vi "From Veristand Master To Modbus.vi"(7 "Parameters":T1={"Interface Data"={"Name"="", "Unit ID"=0, "Refresh Rate"=0, "Write Rate"=0, "Write Mode"=enum."Value Change", "Interface Type"=enum."TCP Master", "TCP Settings"={"Address"="", "Port"=0, "Timeout"=0}, "Serial Settings"={"VISA resource name"="", "baud rate"=0, "parity (even)"=0, "flow control (none)"=0, "serial type"=enum."RTU", "Wire Mode"=-1}}, "Modbus Input Groups"=[], "Modbus Output Groups"=[], "error in (no error)"={"status"=FALSE, "code"=0, "source"=""}, "Modbus Input Engine Group Names"=[], "Modbus Output Engine Group Names"=[]} {"Interface Data"."Serial Settings"."Wire Mode" items=["Unknown"=-1, "RS485/Wire4"=0, "RS485/Wire2-EchoDTR"=1, "RS485/Wire2-CtrlDTR"=2, "RS485/Wire2-Auto"=3, "RS232/DTE"=128, "RS232/DCE"=129, "RS232/AUTO"=130]; "Interface Data"."Serial Settings"."parity (even)" items=["None", "Odd", "Even", "Mark", "Space"]; "Interface Data"."Serial Settings"."flow control (none)" items=["None", "XON/XOFF", "RTS/CTS", "XON/XOFF & RTS/CTS", "DTR/DSR", "XON/XOFF & DTR/DSR"]}, 8 "error in (no error)":errorcluster, 10 "Process in":refnum<class "Process.lvclass">, 11 "Modbus Master in":refnum<class "Modbus Master.lvclass">) -> ()   [LabVIEW 2020, in "Modbus Master Engine.lvlib"]
uses:
  Modbus Master Engine.lvlib
  <vilib>/NI/NIVS Inline Async API/_VS Inline Async API/Process/Process.lvclass
  Shared/Device Info.ctl
  Shared/Write Mode.ctl
  Shared/Controls/Interface Type.ctl
  Shared/Controls/Data Model/TCP Settings.ctl
  Shared/Controls/Data Model/Serial Settings.ctl
  Bulk Data Access.ctl
  System Explorer/SubVIs/Modbus Type.ctl
  Shared/Controls/Data Model/Channel.ctl
  <vilib>/NI VeriStand/Custom Device API/Custom Device Channel Type.ctl
  Shared/Controls/Data Model/Mapping.ctl
  Shared/Controls/Data Model/DataType.ctl
  <vilib>/NI VeriStand/Custom Device API/Custom Device Item Ref.ctl
  Includes/Modbus API.lvlibp/API/Master/Modbus Master.lvclass
  <vilib>/NI/NIVS Inline Async API/_Data Access Engine/Access Type Classes/Read/Read.lvclass/Read.ctl
  <vilib>/NI/NIVS Inline Async API/_VS Inline Async API/Process/Process.lvclass/Process.ctl
  <vilib>/NI/NIVS Inline Async API/_Data Access Engine/Data Access Engine/Methods/Read.Data.vi
  <vilib>/NI/NIVS Inline Async API/_VS Inline Async API/Error Handling Process/SubVIs/Error.ConvertArray.vi
  <vilib>/NI/NIVS Inline Async API/_Data Access Engine/Access Type Classes/Read/Read.ProcessData.vi
  <vilib>/NI/NIVS Inline Async API/_Data Access Engine/Data Access Engine/Data Access Engine.lvclass
  <vilib>/NI VeriStand/Custom Device Tools/Custom Device Utility Library/Custom Device Utility Library.lvlib
  <vilib>/NI/NIVS Inline Async API/_Data Access Engine/Access Type Classes/Write/Write.lvclass
  <vilib>/NI/NIVS Inline Async API/_Data Access Engine/Access Type Classes/Read/Read.lvclass
  Shared/Modbus Master Shared.lvlib
  <vilib>/NI VeriStand/Custom Device API/Custom Device API.lvlib
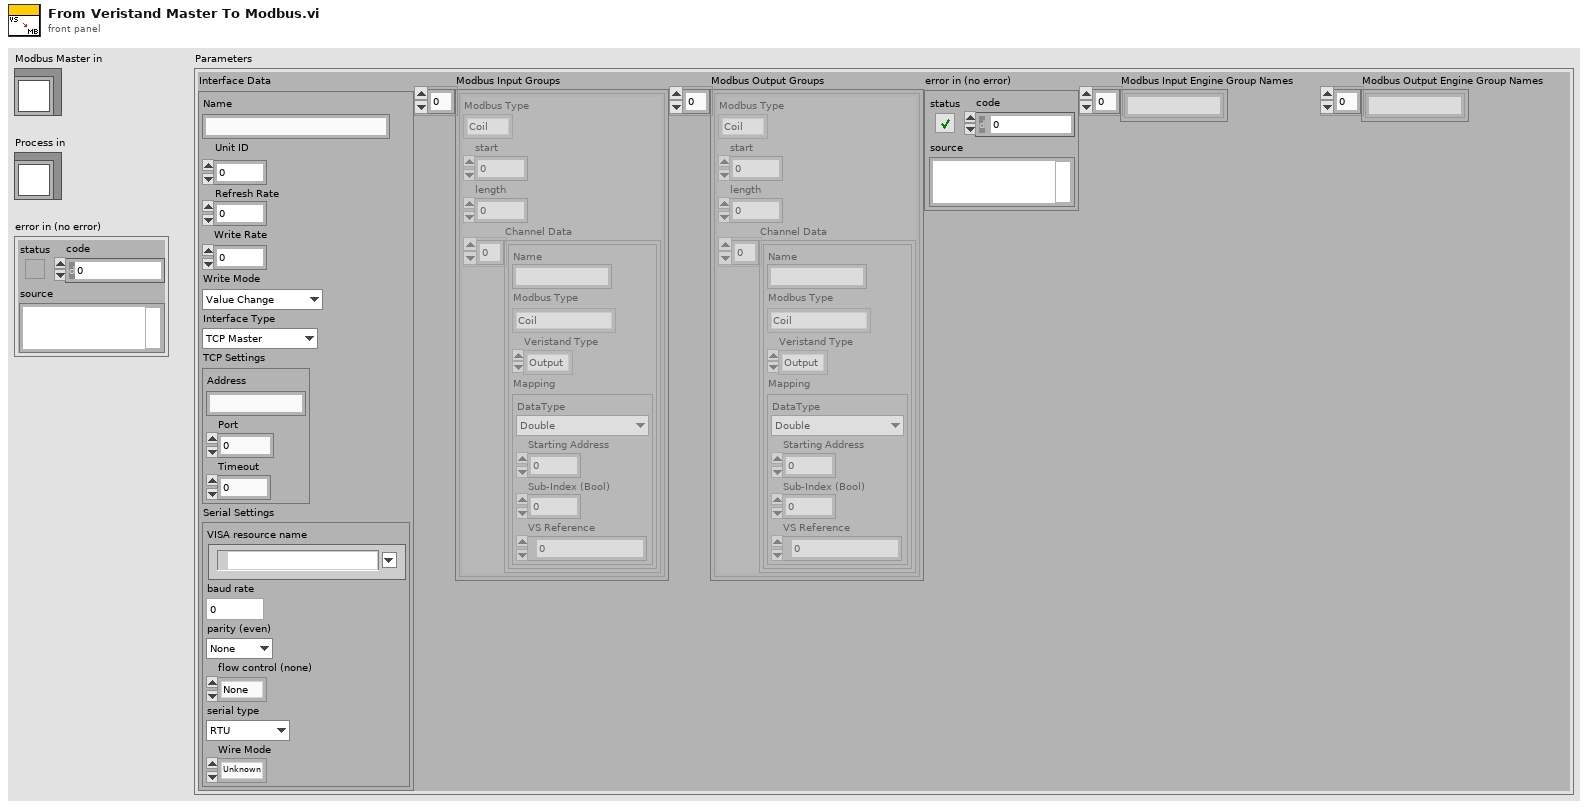
[diagram p1: front panel]
types:
  T1 = typedef "Modbus Master Shared.lvlib/Device Info.ctl" = cluster{"Interface Data":cluster{"Name":string, "Unit ID":u8, "Refresh Rate":i32, "Write Rate":i32, "Write Mode":T2, "Interface Type":T3, "TCP Settings":T4, "Serial Settings":T5}, "Modbus Input Groups":T6[], "Modbus Output Groups":T6[], "error in (no error)":errorcluster, "Modbus Input Engine Group Names":string[], "Modbus Output Engine Group Names":string[]}
  T2 = typedef "Modbus Master Shared.lvlib/Write Mode.ctl" = enum16{"Value Change", "Interval"}
  T3 = typedef "Modbus Master Shared.lvlib/Interface Type.ctl" = enum16{"TCP Master", "Serial Master", "TCP Slave", "Serial Slave"}
  T4 = typedef "Modbus Master Shared.lvlib/TCP Settings.ctl" = cluster{"Address":string, "Port":u16, "Timeout":i32}
  T5 = typedef "Modbus Master Shared.lvlib/Serial Settings.ctl" = cluster{"VISA resource name":refnum<visa-resource-name>, "baud rate":u32, "parity (even)":u16, "flow control (none)":u16, "serial type":enum16{"RTU", "ASCII"}, "Wire Mode":i16}
  T6 = typedef "Modbus Master Shared.lvlib/Bulk Data Access.ctl" = cluster{"Modbus Type":T7, "start":u16, "length":u16, "Channel Data":T8[]}
  T7 = typedef "Modbus Master Shared.lvlib/Modbus Type.ctl" = enum16{"Coil", "Discrete Input", "Holding Register", "Input Register"}
  T8 = typedef "Modbus Master Shared.lvlib/Channel.ctl" = cluster{"Name":string, "Modbus Type":T7, "Veristand Type":T9, "Mapping":T10}
  T9 = typedef "Custom Device API.lvlib/Custom Device Channel Type.ctl" = enum16{"Input", "Output"}
  T10 = typedef "Modbus Master Shared.lvlib/Mapping.ctl" = cluster{"DataType":T11, "Starting Address":u16, "Sub-Index (Bool)":u16, "VS Reference":T12}
  T11 = typedef "Modbus Master Shared.lvlib/DataType.ctl" = enum16{"Double", "Single", "I64", "I32", "I16", "I8", "U64", "U32", "U16", "U8", "Boolean"}
  T12 = typedef "Custom Device API.lvlib/Custom Device Item Ref.ctl" = u64
  T13 = typedef "Data Access Engine.lvlib/Data Access Engine.lvclass/Write.DVR.ctl" = refnum<data-value>
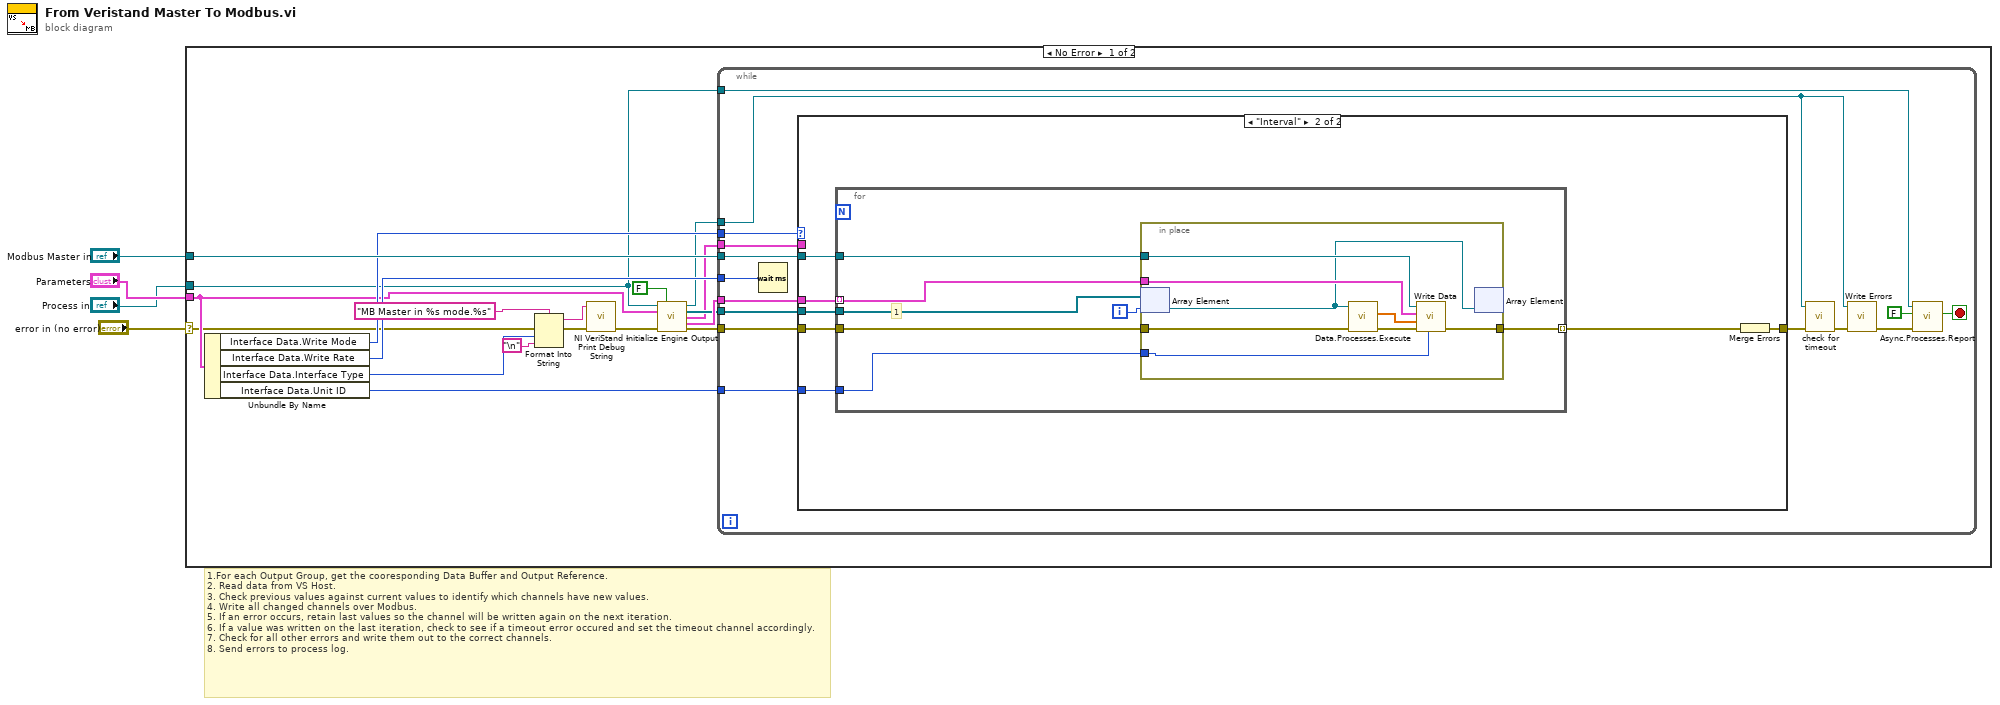
[diagram p0: block diagram]
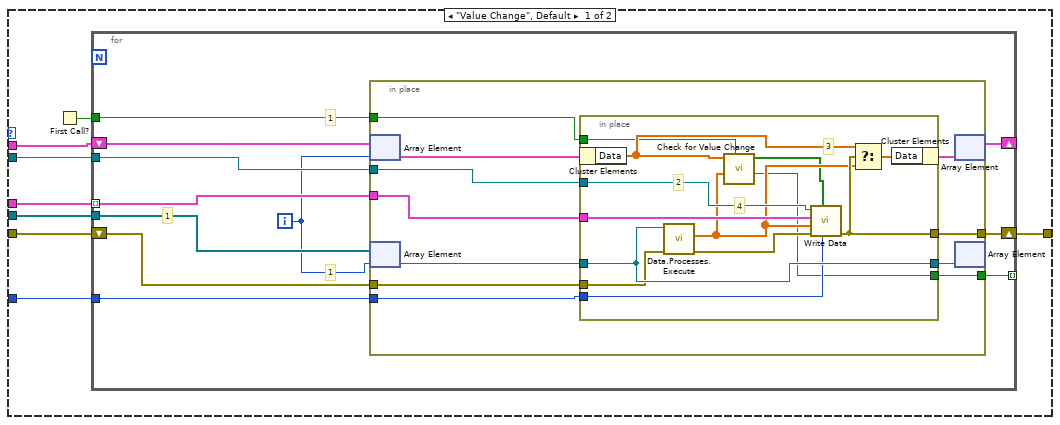
[diagram p2: hidden frame]
diagram:
  # "1.For each Output Group, get the cooresponding Data Buffer and Output Reference.\n2. Read data from VS Host.\n3. Check previous values against current values to identify which channels have new values.\n4. Write all changed channels over Modbus.\n5. If an error occurs, retain last values so the channel will be written again on the next iteration.\n6. If a value was written on the last iteration, check to see if a timeout error occured and set the timeout channel accordingly.\n7. Check for all other errors and write them out to the correct channels.\n8. Send errors to process log."
  n1 = case shown="No Error" "error in (no error)" {
    selector: "error in (no error)" -> [w5 _]
    tunnel: "Parameters" -> [w15 _]
    tunnel: "Modbus Master in" -> [w23 _]
    tunnel: "Process in" -> [w14 _]
    frame No Error {
      n2 = Unbundle By Name(w15) -> ("Interface Data.Write Mode"=w21:T2, "Interface Data.Write Rate"=w22:i32, "Interface Data.Interface Type"=w11:T3, "Interface Data.Unit ID"=w6:u8)
      n3 = Format Into String(format string="MB Master in %s mode.%s", error in=w5, w11, "\n") -> (resulting string=w19:string, error out=w13:errorcluster)  [unwired: 1 in]
      n4 = call <vilib>:"NI VeriStand - Print Debug String.vi"("error in (no error)"=w13, "Message"=w19) -> ("error out"=w20:errorcluster)  [unwired: 9 in]
      n5 = call "Initialize Engine Output.vi"("Process in"=w14, "Init Data Buffers? (T)"=FALSE, "Parameters"=w15, "error in (no error)"=w20) -> ("Diagnostic Group Ref"=w10:T13, "Output Group Refs"=w8:refnum<data-value>[], "Data Buffers"=w7:cluster{"Data":dbl[]}[], "Modbus Output Groups"=w9:T6[], "error out"=w12:errorcluster)  [unwired: 7 in]
      n6 = while {
        tunnel: w14 -> [w38]
        tunnel: w8 -> [w35]
        tunnel: w9 -> [w37]
        tunnel: w23 -> [w36]
        tunnel: w6 -> [w32]
        tunnel: w22 -> [w30]
        tunnel: w10 -> [w26]
        tunnel: w21 -> [w25]
        tunnel: w7 -> [w24]
        tunnel: w12 -> [w31]
        stop <- w34 stop-if-true
        n7 = Wait (ms)(milliseconds to wait=w30) -> ()  [unwired: 1 out]
        n8 = case shown="\"Interval\"" w25 {
          tunnel: w37 -> [w43 w88]
          tunnel: w36 -> [w44 w87]
          tunnel: w35 -> [w42 w86]
          tunnel: w32 -> [w40 w85]
          tunnel: w31 -> [w41 w84]
          tunnel: [w39 w82] -> w28
          tunnel: w24 -> [w45 _]
          frame "Value Change", Default {
            n9 = First Call?() -> (First Call?: T/F=w46:bool)
            n10 = for {
              tunnel: w43 -> [w56] mode=indexing
              tunnel: w44 -> [w57]
              tunnel: w42 -> [w52]
              shift-right: [w53] -> _
              shift-left: w45 -> [w54]
              tunnel: w46 -> [w50]
              tunnel: w40 -> [w49]
              shift-right: [w48] -> w39
              shift-left: w41 -> [w55]
              tunnel: [w47] -> _ mode=indexing
              i -> [w51]
              # "1"
              # "1"
              # "1"
              n11 = in-place {
                in-place-border: w57 -> [w68]
                in-place-border: w56 -> [w67]
                in-place-border: w55 -> [w66]
                in-place-border: [w65] -> w48
                in-place-border: w50 -> [w60]
                in-place-border: w49 -> [w59]
                in-place-border: [w58] -> w47
                n12 = in-place-array #1(w54, w51) -> (w64:cluster{"Data":dbl[]})
                n13 = in-place-array #2(w52, w51) -> (w62:refnum<data-value>)
                n14 = in-place {
                  in-place-border: w68 -> [w79]
                  in-place-border: w67 -> [w76]
                  in-place-border: w66 -> [w80]
                  in-place-border: [w75] -> w65
                  in-place-border: w62 -> [w81]
                  in-place-border: [w81] -> w61
                  in-place-border: w60 -> [w69]
                  in-place-border: w59 -> [w78]
                  in-place-border: [w71] -> w58
                  # "4"
                  # "3"
                  # "2"
                  n15 = in-place-cluster #3(w64) -> ("Data"=w73:dbl[])
                  n16 = call-poly <vilib>:"Data.Processes.Execute.vi"("error in (no error)"=w80, "Ref"=w81) -> ("error out"=w77:errorcluster, "Values"=w72:dbl[])  [unwired: 7 in, 1 out]
                  n17 = call "Check for Value Change.vi"("Force Write?"=w69, "New Data"=w72, "Last Value Data"=w73) -> ("Value Change?"=w71:bool, "Indices to Update"=w70:bool[])  [unwired: 7 in]
                  n18 = call "Write Data.vi"("Unit ID"=w78, "Write Mask"=w70, "error in (no error)"=w77, "Values"=w72, "output data access"=w76, "Modbus Master in"=w79) -> ("error out"=w75:errorcluster)  [unwired: 5 in]
                  n19 = Select(t=w73, s=w75, f=w72) -> (s? t:f=w74:dbl[])
                  n20 = in-place-cluster #3("Data"=w74) -> (w63:cluster{"Data":dbl[]})
                }
                n21 = in-place-array #1(w63) -> (w53:cluster{"Data":dbl[]}[])  [unwired: 1 out]
                n22 = in-place-array #2(w61) -> ()  [unwired: 2 out]
              }
            }
          }
          frame "Interval" {
            n23 = for {
              tunnel: w88 -> [w94] mode=indexing
              tunnel: w87 -> [w95]
              tunnel: w86 -> [w92]
              tunnel: w85 -> [w90]
              tunnel: w84 -> [w93]
              tunnel: [w89] -> w83 mode=indexing
              i -> [w91]
              # "1"
              n24 = in-place {
                in-place-border: w95 -> [w103]
                in-place-border: w94 -> [w102]
                in-place-border: w93 -> [w101]
                in-place-border: [w100] -> w89
                in-place-border: w90 -> [w98]
                n25 = in-place-array #4(w92, w91) -> (w99:refnum<data-value>)
                n26 = call-poly <vilib>:"Data.Processes.Execute.vi"("error in (no error)"=w101, "Ref"=w99) -> ("error out"=w97:errorcluster, "Values"=w96:dbl[])  [unwired: 7 in, 1 out]
                n27 = call "Write Data.vi"("Unit ID"=w98, "error in (no error)"=w97, "Values"=w96, "output data access"=w102, "Modbus Master in"=w103) -> ("error out"=w100:errorcluster)  [unwired: 6 in]
                n28 = in-place-array #4(w99) -> ()  [unwired: 2 out]
              }
            }
            n29 = Merge Errors(w83) -> (w82:errorcluster)
          }
        }
        n30 = call "check for timeout.vi"("error in (no error)"=w28, "Data Value Reference in"=w26) -> ("error out"=w27:errorcluster)  [unwired: 9 in]
        n31 = call "Write Errors.vi"("error in (no error)"=w27, "Data Value Reference in"=w26) -> ("error out"=w29:errorcluster)  [unwired: 9 in]
        n32 = call <vilib>:"Async.Processes.Report.vi"("Error"=w29, "Stop Async on Error?"=FALSE ("Stop on Error?"), "Process in"=w38) -> ("Stop"=w34:bool)  [unwired: 7 in, 1 out]
      }
    }
    frame Error {
    }
  }
